vi "GageAdvancedwithFreq Doubler.vi"(6 "Enum":T1(ring)=enum."Quadrupled Frequency", 8 "Clock Gen Params":T2={"low cuttoff"=8000000.0, "high cutoff"=12000000.0, "trimmed length"=14800, "front-end samples"=400, "duty cycle (fract)"=0.6, "Gage output channel"=1}, 9 "Gage Speed":dbl(ring)=1000000000.0 items=["Slow Gage"=300000000.0, "Fast Gage"=1000000000.0], 10 "Sweep Speed":dbl=20000.0, 11 "k-space signal in":u16[](array[numeric])=array[5000 elements]) -> (3 "final waveform generated":u16[](graph))   [LabVIEW 2012]
uses:
  <vilib>/Analysis/NI_AALPro.lvlib
  <vilib>/Analysis/2dsp.llb/Real FFT.vi
  <vilib>/Analysis/NI_AALBase.lvlib
  <vilib>/Analysis/3filter.llb/Butterworth Filter (DBL).vi
  <vilib>/Analysis/3filter.llb/Zero Phase Filter (obs, DBL).vi
  <vilib>/measure/NI_MAPro.lvlib
  <vilib>/measure/maspectr.llb/FFT Power Spectrum and PSD for 1 Chan.vi
  <vilib>/measure/maresamp.llb/Resample Waveform (continuous).vi
panel:
  out "pre-upsample PSD":cluster{"f0":dbl, "df":dbl, "magnitude":dbl[]}[](graph)
  out "size(s) 2":i32
  out "upsample PSD":cluster{"f0":dbl, "df":dbl, "magnitude":dbl[]}[](graph)
  out "result":dbl
  out "Doubled Freq":dbl[](array[numeric])
  out "duty cycle (fract)":sgl=0.6
  out "Number of Points per clock sweep - 5%":dbl=47500.0
  out "No Freq Modifications":dbl[](array[numeric])
  out "low cuttoff":dbl=1000000.0
  out "high cutoff":dbl=45000000.0
  out "final waveform generated 2":dbl[][](graph)
  out "size(s)":i32=8800
  out "Freq domain (raw and filtered)":dbl[][](graph)
  out "Time domain (raw and filtered)":dbl[](graph)
  out "Channels Found":i32=1
  out "Board Name":string="CG11G"
  out "Boards Found":i32=1
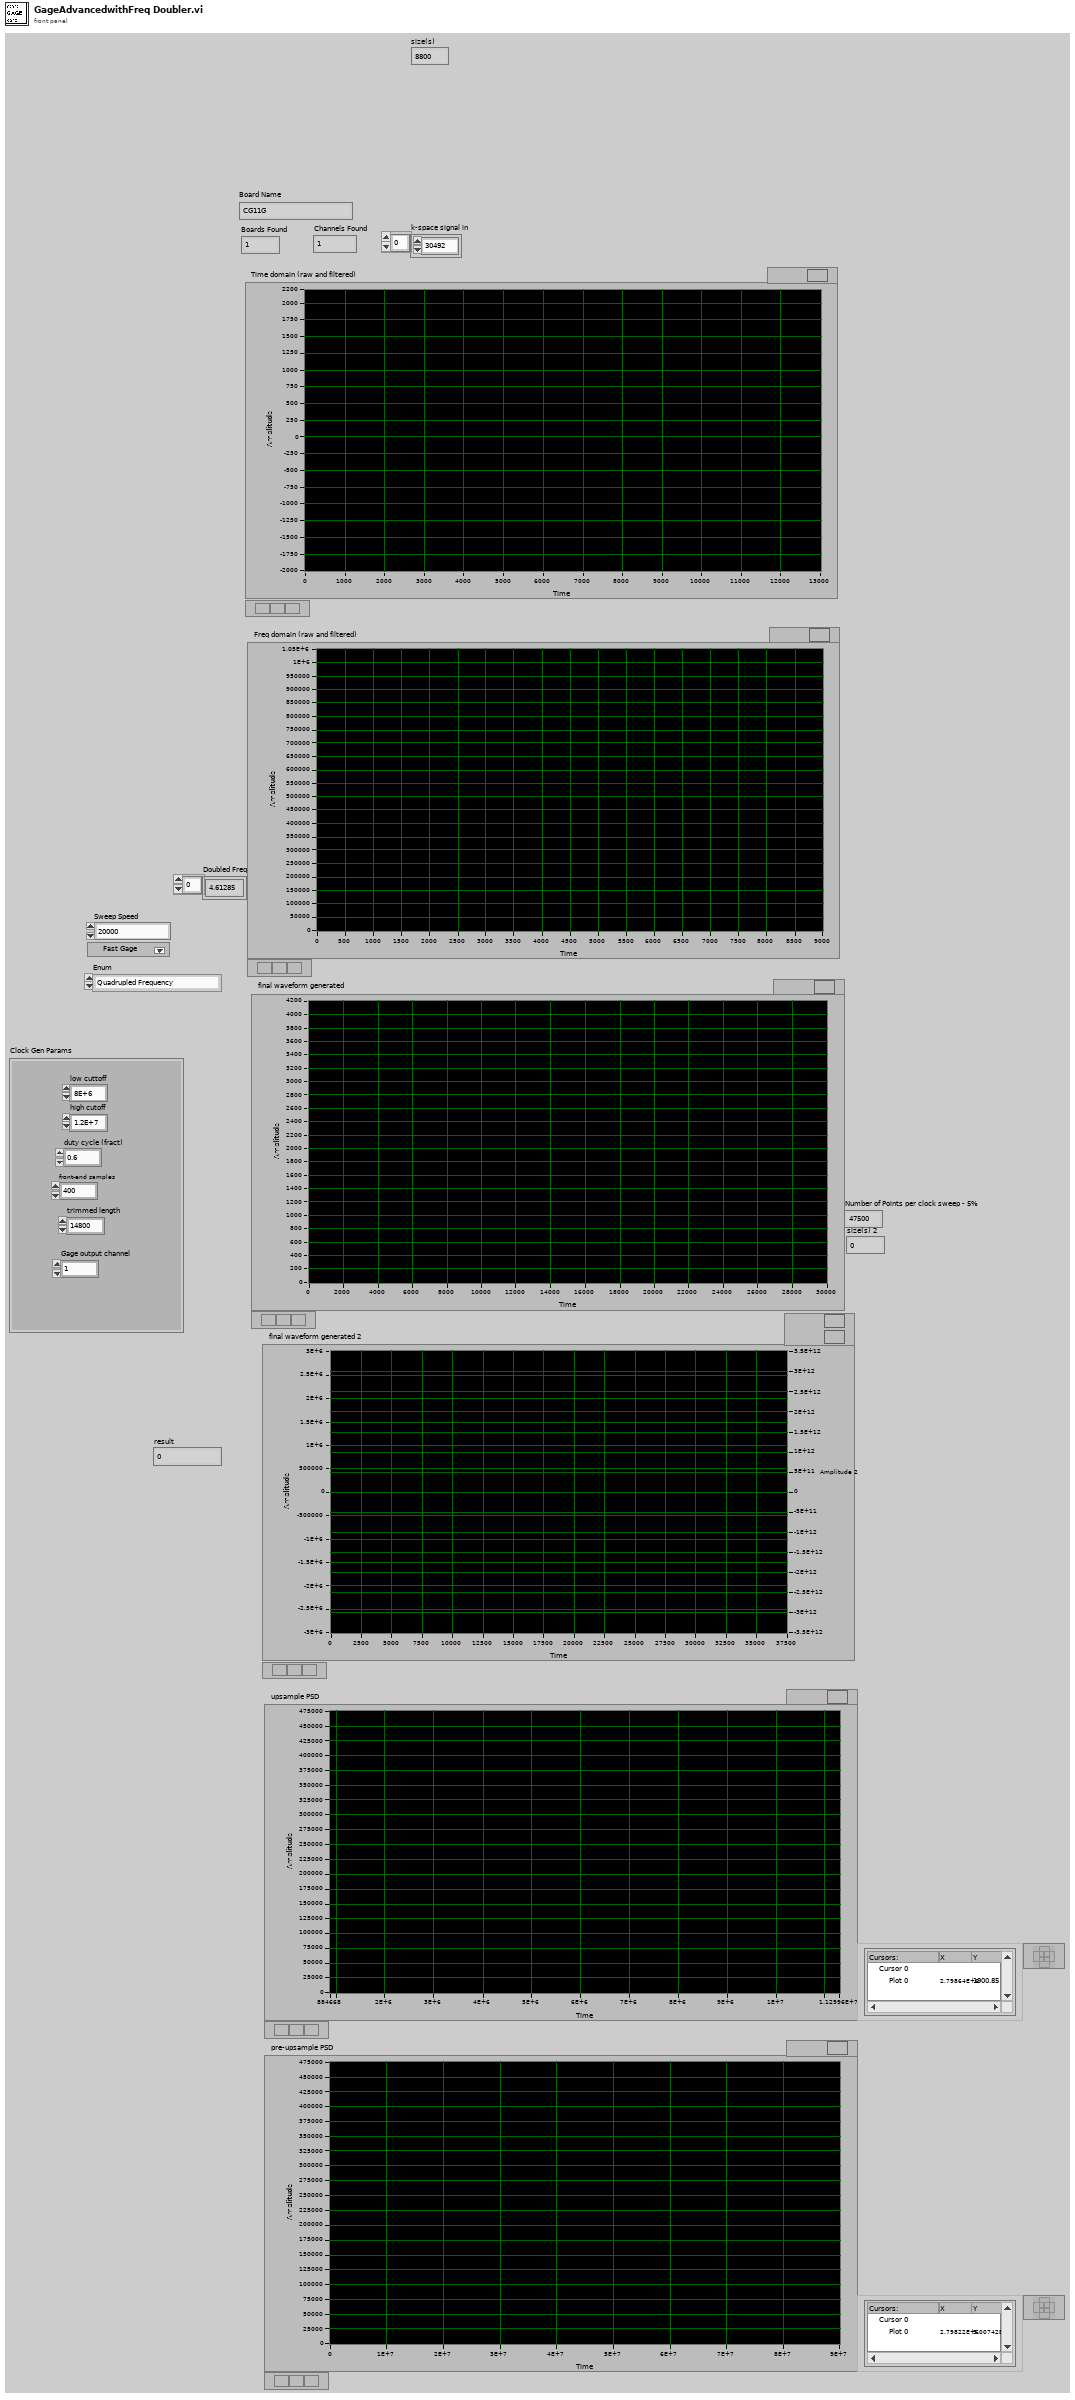
[diagram p1: front panel]
types:
  T1 = enum16{"No Frequency Enhancement", "Doubled Frequency", "Quadrupled Frequency"}
  T2 = cluster{"low cuttoff":dbl, "high cutoff":dbl, "trimmed length":i32, "front-end samples":i32, "duty cycle (fract)":sgl, "Gage output channel":i32}
  T3 = enum32{"Lowpass", "Highpass", "Bandpass", "Bandstop"}
  T4 = cluster{"filter structure":enum32{"IIR 2nd Order", "IIR 4th Order"}, "Reverse Coefficients":dbl[], "Forward Coefficients":dbl[]}
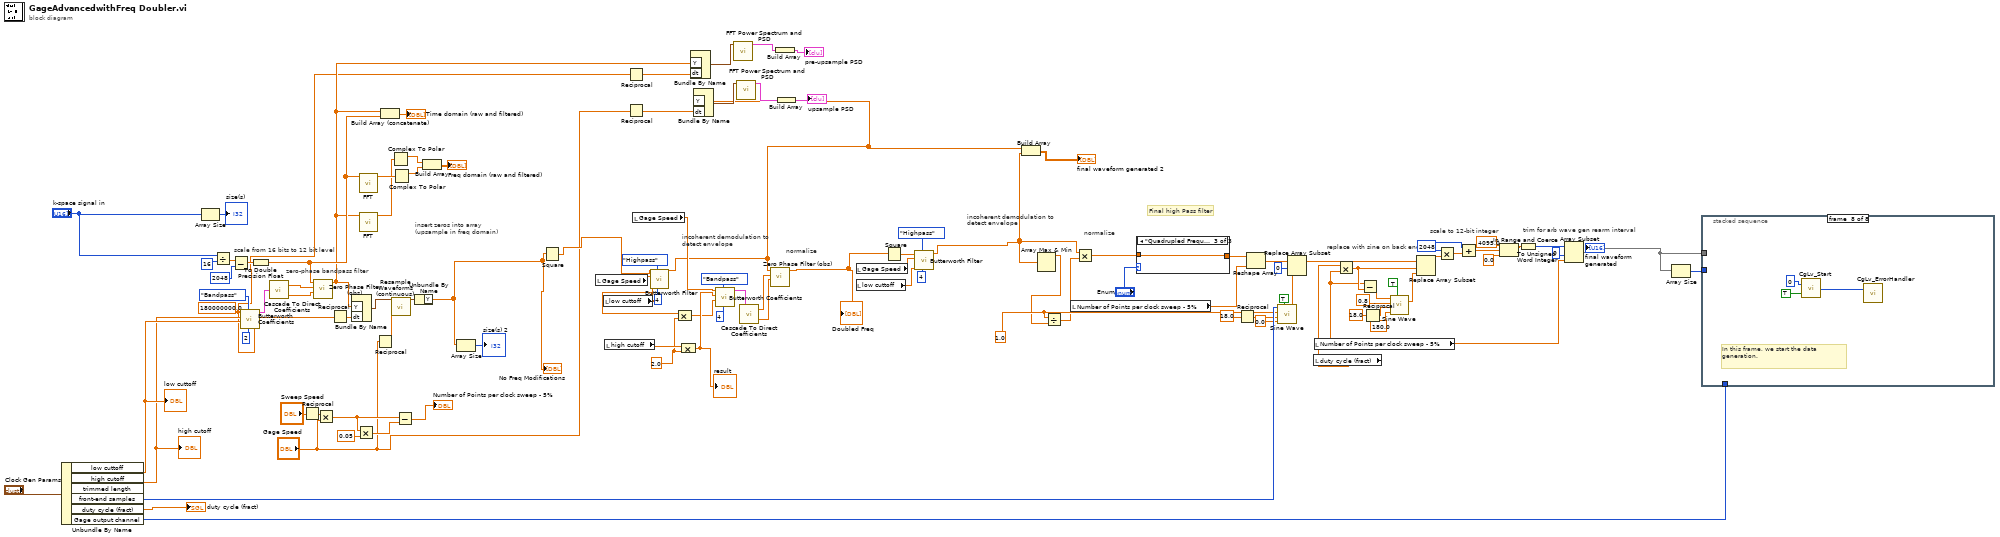
[diagram p0: block diagram]
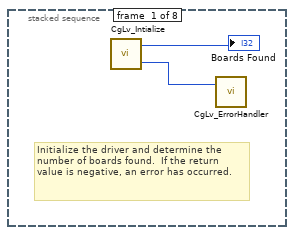
[diagram p2: hidden frame]
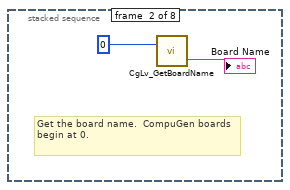
[diagram p3: hidden frame]
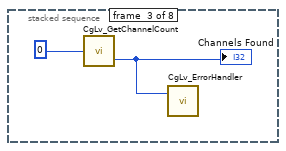
[diagram p4: hidden frame]
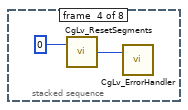
[diagram p5: hidden frame]
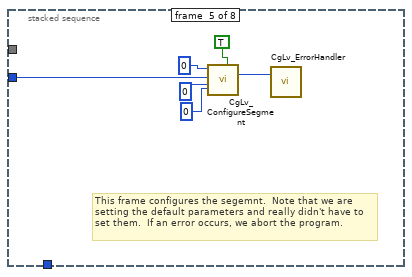
[diagram p6: hidden frame]
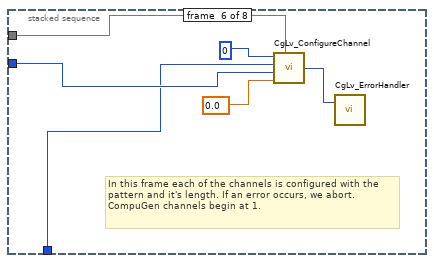
[diagram p7: hidden frame]
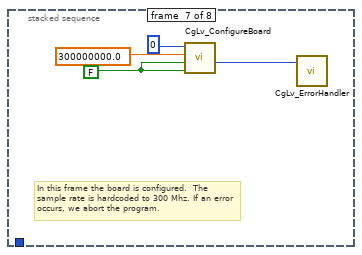
[diagram p8: hidden frame]
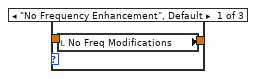
[diagram p9: hidden frame]
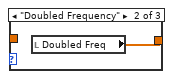
[diagram p10: hidden frame]
diagram:
  w58 = i16 2048 ("n")
  w6 = 1.0 ("amplitude")
  w29 = 2.0 ("y")
  w17 = 180000000.0 ("sampling freq: fs")
  # "trim for arb wave gen rearm interval"
  # "scale to 12-bit integer"
  # "replace with sine on back end"
  # "Final high Pass filter"
  # "normalize"
  # "incoherent demodulation to\ndetect envelope"
  # "normalize"
  # "incoherent demodulation to\ndetect envelope"
  # "scale from 16 bits to 12 bit level"
  # "insert zeros into array\n(upsample in freq domain)"
  # "zero-phase bandpass filter"
  n1 = Unbundle By Name("Clock Gen Params") -> ("low cuttoff"=w81:dbl, "high cutoff"=w80:dbl, "front-end samples"=w93:i32, "duty cycle (fract)"=→"duty cycle (fract)":sgl, "Gage output channel"=w91:i32)  [unwired: 1 out]
  "high cutoff" <- w80
  "low cuttoff" <- w81
  n2 = Array Size(array="k-space signal in") -> (size(s)=→"size(s)":i32)
  n3 = Divide(x="k-space signal in", y=i16 16 ("n")) -> (x/y=w105:dbl[])
  n4 = Subtract(x=w105, y=i16 2048 ("n")) -> (x-y=w95:dbl[])
  n5 = call <vilib>:"Butterworth Coefficients.vi"("order"=2, "filter type"=T3."Bandpass", "low cutoff freq: fl"=w81, "high cutoff freq: fh"=w80, "sampling freq: fs"=w17) -> ("IIR Filter Cluster"=w42:T4)  [unwired: 5 in, 1 out]
  n6 = To Double Precision Float(number=w95) -> (double precision float=w39:dbl[])
  n7 = call <vilib>:"Cascade To Direct Coefficients.vi"("IIR Filter Cluster"=w42) -> ("Reverse Coefficients"=w41:dbl[], "Forward Coefficients"=w40:dbl[])
  n8 = Reciprocal(x="Sweep Speed") -> (1/x=w86:dbl)
  n9 = call-poly <vilib>:"Zero Phase Filter (obs).vi"("Forward Coefficients"=w40, "Reverse Coefficients"=w41, "X"=w39) -> ("Filtered X"=w18:dbl[])  [unwired: 7 in, 1 out]
  n10 = Multiply(x=w86, y="Gage Speed") -> (x*y=w19:dbl)
  n11 = Reciprocal(x=w17) -> (1/x=w16:dbl)
  n12 = Bundle By Name("Y"=w18, "dt"=w16) -> (w15:waveform(dbl))  [unwired: 1 in]
  n13 = Multiply(x=w19, y=0.05) -> (x*y=w82:dbl)
  n14 = call-poly <vilib>:"FFT.vi"("X"=w39) -> ("FFT {X}"=w96:cdb[])  [unwired: 9 in, 1 out]
  n15 = call-poly <vilib>:"FFT.vi"("X"=w18) -> ("FFT {X}"=w20:cdb[])  [unwired: 9 in, 1 out]
  n16 = Reciprocal(x="Gage Speed") -> (1/x=w13:dbl)
  n17 = Build Array (concatenate)(w18, w39) -> (→"Time domain (raw and filtered)":dbl[])
  n18 = call-poly <vilib>:"Resample Waveforms (continuous).vi"("waveform in"=w15, "dt"=w13) -> ("resampled waveform out"=w12:waveform(dbl))  [unwired: 9 in, 4 out]
  n19 = Complex To Polar(r * e^(i*theta)=w20) -> (r=w102:dbl[])  [unwired: 1 out]
  n20 = Complex To Polar(r * e^(i*theta)=w96) -> (r=w103:dbl[])  [unwired: 1 out]
  n21 = Subtract(x=w19, y=w82) -> (x-y=→"Number of Points per clock sweep - 5%":dbl)
  n22 = Unbundle By Name(w12) -> ("Y"=w10:dbl[])
  "No Freq Modifications" <- w10
  n23 = Build Array(w102, w103) -> (→"Freq domain (raw and filtered)":dbl[][])
  n24 = Array Size(array=w10) -> (size(s)=→"size(s) 2":i32)
  n25 = Square(x=w10) -> (x^2=w27:dbl[])
  n26 = local read "Gage Speed"() -> (w79:dbl)
  n27 = local read "low cuttoff"() -> (w30:dbl)
  n28 = local read "high cutoff"() -> (w33:dbl)
  n29 = Reciprocal(x=w17) -> (1/x=w24:dbl)
  n30 = Reciprocal(x="Gage Speed") -> (1/x=w34:dbl)
  n31 = local read "Gage Speed"() -> (w78:dbl)
  n32 = call-poly <vilib>:"Butterworth Filter.vi"("order"=4, "filter type"=T3."Highpass", "low cutoff freq: fl"=w30, "sampling freq: fs"=w79, "X"=w27) -> ("Filtered X"=w9:dbl[])  [unwired: 3 in, 1 out]
  n33 = Compound Arithmetic op=MULTIPLY(w30, w29) -> (w28:dbl)
  n34 = Compound Arithmetic op=MULTIPLY(w33, w29) -> (w31:dbl)
  "result" <- w31
  n35 = Bundle By Name("Y"=w18, "dt"=w24) -> (w25:waveform(dbl))  [unwired: 1 in]
  n36 = Bundle By Name("Y"=w9, "dt"=w34) -> (w11:waveform(dbl))  [unwired: 1 in]
  n37 = call <vilib>:"Butterworth Coefficients.vi"("order"=4, "filter type"=T3."Bandpass", "low cutoff freq: fl"=w28, "high cutoff freq: fh"=w31, "sampling freq: fs"=w78) -> ("IIR Filter Cluster"=w38:T4)  [unwired: 5 in, 1 out]
  n38 = call-poly <vilib>:"FFT Power Spectrum and PSD.vi"("time signal"=w25) -> ("Power Spectrum / PSD"=w22:cluster{"f0":dbl, "df":dbl, "magnitude":dbl[]})  [unwired: 7 in, 3 out]
  n39 = call-poly <vilib>:"FFT Power Spectrum and PSD.vi"("time signal"=w11) -> ("Power Spectrum / PSD"=w23:cluster{"f0":dbl, "df":dbl, "magnitude":dbl[]})  [unwired: 7 in, 3 out]
  n40 = call <vilib>:"Cascade To Direct Coefficients.vi"("IIR Filter Cluster"=w38) -> ("Reverse Coefficients"=w37:dbl[], "Forward Coefficients"=w36:dbl[])
  n41 = call-poly <vilib>:"Zero Phase Filter (obs).vi"("Forward Coefficients"=w36, "Reverse Coefficients"=w37, "X"=w9) -> ("Filtered X"=w8:dbl[])  [unwired: 7 in, 1 out]
  "Doubled Freq" <- w8
  n42 = Build Array(w22) -> (→"pre-upsample PSD":cluster{"f0":dbl, "df":dbl, "magnitude":dbl[]}[])
  n43 = Build Array(w23) -> (→"upsample PSD":cluster{"f0":dbl, "df":dbl, "magnitude":dbl[]}[])
  n44 = local read "Gage Speed"() -> (w76:dbl)
  n45 = local read "low cuttoff"() -> (w75:dbl)
  n46 = Square(x=w8) -> (x^2=w7:dbl[])
  n47 = call-poly <vilib>:"Butterworth Filter.vi"("order"=4, "filter type"=T3."Highpass", "low cutoff freq: fl"=w75, "sampling freq: fs"=w76, "X"=w7) -> ("Filtered X"=w3:dbl[])  [unwired: 3 in, 1 out]
  n48 = Build Array(w9, w3) -> (→"final waveform generated 2":dbl[][])
  n49 = Array Max & Min(array=w3) -> (max value=w5:dbl)  [unwired: 3 out]
  n50 = Divide(x=w6, y=w5) -> (x/y=w4:dbl)
  n51 = local read "Number of Points per clock sweep - 5%"() -> (w48:dbl)
  n52 = Multiply(x=w3, y=w4) -> (x*y=w2:dbl[])
  n53 = case shown="\"Quadrupled Frequency\"" "Enum" {
    tunnel: [w108 w109 w110] -> w46
    tunnel: w2 -> [_ _ w110]
    frame "No Frequency Enhancement", Default {
      n54 = local read "No Freq Modifications"() -> (w108:dbl[])
    }
    frame "Doubled Frequency" {
      n55 = local read "Doubled Freq"() -> (w109:dbl[])
    }
    frame "Quadrupled Frequency" {
    }
  }
  n56 = Reciprocal(x=18.0 ("amplitude")) -> (1/x=w68:dbl)
  n57 = Reshape Array(w46, w48) -> (w47:dbl[])
  n58 = call <vilib>:"Sine Wave.vi"("samples"=w93, "amplitude"=w6, "frequency"=w68, "phase in"=0.0, "reset phase"=TRUE) -> ("sine wave"=w69:dbl[])  [unwired: 2 out]
  n59 = Replace Array Subset(array=w47, new element=w69, index=0) -> (w61:dbl[])
  n60 = local read "duty cycle (fract)"() -> (w44:sgl)
  n61 = local read "Number of Points per clock sweep - 5%"() -> (w45:dbl)
  n62 = Multiply(x=w44, y=w45) -> (x*y=w53:dbl)
  n63 = Subtract(x=w45, y=w53) -> (x-y=w54:dbl)
  n64 = Reciprocal(x=18.0 ("amplitude")) -> (1/x=w65:dbl)
  n65 = call <vilib>:"Sine Wave.vi"("samples"=w54, "amplitude"=0.8, "frequency"=w65, "phase in"=180.0, "reset phase"=TRUE) -> ("sine wave"=w60:dbl[])  [unwired: 2 out]
  n66 = Replace Array Subset(array=w61, new element=w60, index=w53) -> (w49:dbl[])
  n67 = Multiply(x=w58, y=w49) -> (x*y=w59:dbl[])
  n68 = Add(x=w58, y=w59) -> (x+y=w50:dbl[])
  n69 = In Range and Coerce(upper limit=sgl 4095.0 ("n"), x=w50, lower limit=sgl 0.0 ("n")) -> (coerced(x)=w51:dbl[])  [unwired: 1 out]
  n70 = To Unsigned Word Integer(number=w51) -> (unsigned 16bit integer=w57:u16[])
  n71 = Array Subset(array=w57, index=0, length=w45) -> (w52:u16[])
  "final waveform generated" <- w52
  n72 = Array Size(array=w52) -> (size(s)=w43:i32)
  n73 = stacked-sequence {
    tunnel: w52 -> [_ _ _ _ _ w127 _ _]
    tunnel: w43 -> [_ _ _ _ w119 w126 _ _]
    tunnel: w91 -> [_ _ _ _ _ w125 _ _]
    frame #0 {
      # "Initialize the driver and determine the number of boards found.  If the return value is negative, an error has occurred."
      n74 = call "CgLv_Intialize.vi"() -> ("Error Code"=w111:i32, "Boards Found"=→"Boards Found":i32)
      n75 = call "CgLv_ErrorHandler.vi"("Error Code"=w111) -> ()  [unwired: 1 in, 1 out]
    }
    frame #1 {
      # "Get the board name.  CompuGen boards begin at 0."
      n76 = call "CgLv_GetBoardName.vi"("Board Number"=u32 0) -> ("Board Name"=→"Board Name":string)  [unwired: 1 out]
    }
    frame #2 {
      n77 = call "CgLv_GetChannelCount.vi"("Board Number"=u32 0) -> ("Channels"=w115:i32)  [unwired: 1 out]
      "Channels Found" <- w115
      n78 = call "CgLv_ErrorHandler.vi"("Error Code"=w115) -> ()  [unwired: 1 in, 1 out]
    }
    frame #3 {
      n79 = call "CgLv_ResetSegments.vi"("Board Number (0)"=0) -> ("Error Code"=w117:i32)  [unwired: 1 in]
      n80 = call "CgLv_ErrorHandler.vi"("Error Code"=w117) -> ()  [unwired: 1 in, 1 out]
    }
    frame #4 {
      # "This frame configures the segemnt.  Note that we are setting the default parameters and really didn't have to set them.  If an error occurs, we abort the program."
      n81 = call "CgLv_ConfigureSegment.vi"("Triggered (f)"=TRUE ("Ext Triggered?"), "Marker (0)"=u32 0 ("Marker position"), "Loop Count (0)"=u32 0, "Length (1024)"=w119, "Board Number (0)"=u32 0) -> ("Error Code"=w122:i32)  [unwired: 6 in]
      n82 = call "CgLv_ErrorHandler.vi"("Error Code"=w122) -> ()  [unwired: 1 in, 1 out]
    }
    frame #5 {
      # "In this frame each of the channels is configured with the pattern and it's length. If an error occurs, we abort.  CompuGen channels begin at 1."
      n83 = call "CgLv_ConfigureChannel.vi"("Board Number (0)"=u32 0, "Channel Number (1)"=w125, "Buffer Length (1024)"=w126, "Attenuation (0)"=sgl 0.0, "Buffer"=w127) -> ("Error Code"=w128:i32)
      n84 = call "CgLv_ErrorHandler.vi"("Error Code"=w128) -> ()  [unwired: 1 in, 1 out]
    }
    frame #6 {
      w133 = FALSE
      # "In this frame the board is configured.  The sample rate is hardcoded to 300 Mhz. If an error occurs, we abort the program."
      n85 = call "CgLv_ConfigureBoard.vi"("Reserved (f)"=w133, "External Clock (f)"=w133, "Conversion Rate (150 MHz)"=sgl 300000000.0, "Board Number (0)"=0) -> ("Error Code"=w132:i32)
      n86 = call "CgLv_ErrorHandler.vi"("Error Code"=w132) -> ()  [unwired: 1 in, 1 out]
    }
    frame #7 {
      # "In this frame, we start the data generation."
      n87 = call "CgLv_Start.vi"("Triggered (f)"=TRUE, "Board Number (0)"=u32 0) -> ("Error Code"=w136:i32)
      n88 = call "CgLv_ErrorHandler.vi"("Error Code"=w136) -> ()  [unwired: 1 in, 1 out]
    }
  }
